vi "populate.vi"(0 "ILCFactory in":refnum<class "ILCFactory.lvclass">, 5 "ILC in":refnum<class "ILC.lvclass">, 7 "Settings":T2, 9 "Timings":T1, 11 "error in (no error)":errorcluster) -> (4 "ILCFactory out":refnum<class "ILCFactory.lvclass">, 6 "ILC out":refnum<class "ILC.lvclass">, 15 "error out":errorcluster)   [LabVIEW 2016, in "RTILC.lvlib" / "ILCFactory.lvclass"]
uses:
  ILCFactory.lvclass
  DataTypes/ILCSettings.ctl
  ILC/ILC.lvclass
  DataTypes/ILCTimings.ctl
  DataTypes/ILCData.ctl
  DataTypes/ILCConstants.ctl
  DataTypes/ILCCommand.ctl
  DataTypes/ILCScanRates.ctl
  DataTypes/ILCTelemetry.ctl
  DataTypes/ILCResponses.ctl
  Common_RT_Modbus/DataTypes/ExceptionCodes.ctl
  ILC/ILC.lvclass/ILC.ctl
  RTILC.lvlib
  Common_RT_Modbus/RTModbus.lvlib
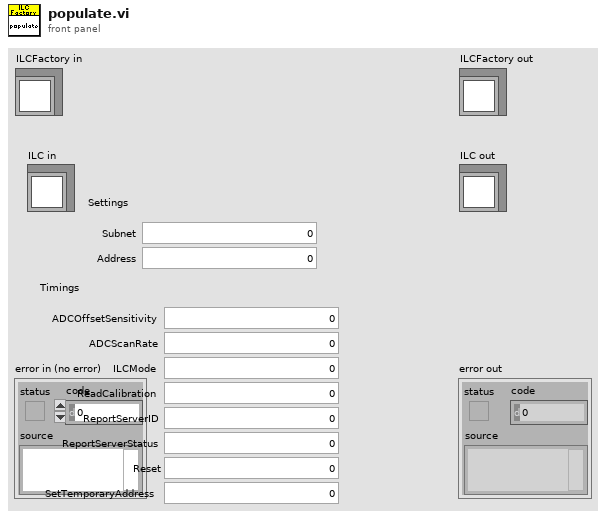
[diagram p1: front panel]
types:
  T1 = typedef "RTILC.lvlib/ILCTimings.ctl" = cluster{"ADCOffsetSensitivity":u32, "ADCScanRate":u32, "ILCMode":u32, "ReadCalibration":u32, "ReportServerID":u32, "ReportServerStatus":u32, "Reset":u32, "SetTemporaryAddress":u32}
  T2 = typedef "RTILC.lvlib/ILCSettings.ctl" = cluster{"Subnet":u8, "Address":u8}
  T3 = typedef "RTILC.lvlib/ILCData.ctl" = cluster{"Constants":T4, "Command":T5, "Telemetry":T7, "Responses":T8, "Timings":T1}
  T4 = typedef "RTILC.lvlib/ILCConstants.ctl" = cluster{"Subnet":u8, "Address":u8}
  T5 = typedef "RTILC.lvlib/ILCCommand.ctl" = cluster{"ILCMode":u16, "TemporaryAddress":u8, "ADCScanRate":T6, "ADCChannel":u8, "ADCOffset":sgl, "ADCSensitivity":sgl}
  T6 = typedef "RTILC.lvlib/ILCScanRates.ctl" = u8
  T7 = typedef "RTILC.lvlib/ILCTelemetry.ctl" = cluster{"UniqueID":u64, "FirmwareType":u8, "NetworkNodeType":u8, "ILCOption":u8, "NetworkNodeOption":u8, "MajorRevision":u8, "MinorRevision":u8, "FirmwareName":string, "ILCMode":u16, "MajorFault":bool, "MinorFault":bool, "FaultOverride":bool, "UniqueIDCRCMismatch":bool, "AppTypeNodeTypeMismatch":bool, "AppMissing":bool, "AppCRCMismatch":bool, "TEDSNotFound":bool, "TEDS1Mismatch":bool, "TEDS2Mismatch":bool, "WatchdogResetDetected":bool, "BrownoutDetected":bool, "EventTrapResetDetected":bool, "TemporaryAddress":u8, "ADCScanRate":T6, "DAC1":u16, "DAC2":u16, "DAC3":u16, "DAC4":u16, "MainADCCalibrationK":sgl[], "MainSensorOffset":sgl[], "MainSensorSensitivity":sgl[], "BackupADCCalibrationK":sgl[], "BackupSensorOffset":sgl[], "BackupSensorSensitivity":sgl[]}
  T8 = typedef "RTILC.lvlib/ILCResponses.ctl" = cluster{"ReportServerID":T9, "ReportServerStatus":T9, "ILCMode":T9, "SetTemporaryAddress":T9, "Reset":T9, "ADCScanRate":T9, "ADCOffsetSensitivity":T9, "ReadDAC":T9, "ReadCalibration":T9}
  T9 = typedef "RTModbus.lvlib/ExceptionCodes.ctl" = u16
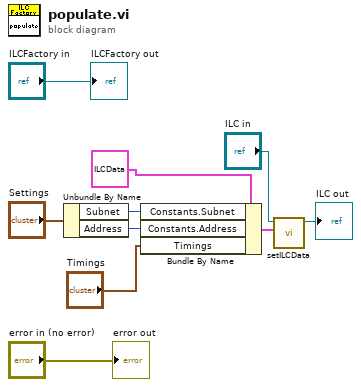
[diagram p0: block diagram]
diagram:
  n1 = Unbundle By Name("Settings") -> ("Subnet"=w8:u8, "Address"=w7:u8)
  n2 = Bundle By Name(cluster=T3 {"Constants"={"Subnet"=0, "Address"=0}, "Command"={"ILCMode"=0, "TemporaryAddress"=0, "ADCScanRate"=0, "ADCChannel"=0, "ADCOffset"=0.0, "ADCSensitivity"=0.0}, "Telemetry"={"UniqueID"=0, "FirmwareType"=0, "NetworkNodeType"=0, "ILCOption"=0, "NetworkNodeOption"=0, "MajorRevision"=0, "MinorRevision"=0, "FirmwareName"="", "ILCMode"=0, "MajorFault"=FALSE, "MinorFault"=FALSE, "FaultOverride"=FALSE, "UniqueIDCRCMismatch"=FALSE, "AppTypeNodeTypeMismatch"=FALSE, "AppMissing"=FALSE, "AppCRCMismatch"=FALSE, "TEDSNotFound"=FALSE, "TEDS1Mismatch"=FALSE, "TEDS2Mismatch"=FALSE, "WatchdogResetDetected"=FALSE, "BrownoutDetected"=FALSE, "EventTrapResetDetected"=FALSE, "TemporaryAddress"=0, "ADCScanRate"=0, "DAC1"=0, "DAC2"=0, "DAC3"=0, "DAC4"=0, "MainADCCalibrationK"=[], "MainSensorOffset"=[], "MainSensorSensitivity"=[], "BackupADCCalibrationK"=[], "BackupSensorOffset"=[], "BackupSensorSensitivity"=[]}, "Responses"={"ReportServerID"=0, "ReportServerStatus"=0, "ILCMode"=0, "SetTemporaryAddress"=0, "Reset"=0, "ADCScanRate"=0, "ADCOffsetSensitivity"=0, "ReadDAC"=0, "ReadCalibration"=0}, "Timings"={"ADCOffsetSensitivity"=0, "ADCScanRate"=0, "ILCMode"=0, "ReadCalibration"=0, "ReportServerID"=0, "ReportServerStatus"=0, "Reset"=0, "SetTemporaryAddress"=0}} ("ILCData"), "Constants.Subnet"=w8, "Constants.Address"=w7, "Timings"="Timings") -> (w6:T3)
  n3 = call "setILCData.vi"("ILCData"=w6, "ILC in"="ILC in") -> ("ILC out"=→"ILC out":refnum<class "ILC.lvclass">)  [unwired: 9 in]
  "error out" <- "error in (no error)"
  "ILCFactory out" <- "ILCFactory in"
